vi "insert new subpanel.vi"(8 "error in":errorcluster, 9 "event":refnum<user-event>, 10 "mod data ref":refnum<data-value>, 11 "SubPanel in":refnum<vi>) -> (0 "error out":errorcluster, 3 "reference out":refnum<vi>)   [LabVIEW 2013, in "vi mod UI.lvlib"]
uses:
  vi mod UI.lvlib
  VI modification.lvclass
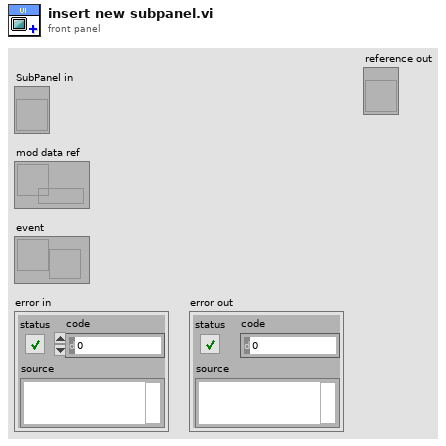
[diagram p1: front panel]
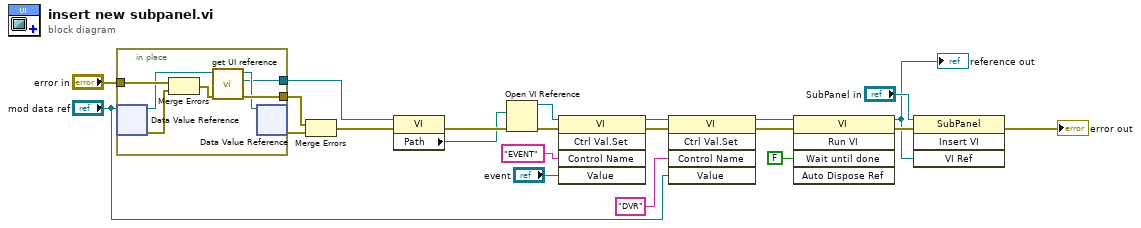
[diagram p0: block diagram]
diagram:
  n1 = in-place {
    in-place-border: "error in" -> [w29]
    in-place-border: [w28] -> w20
    in-place-border: [w23] -> w5
    n2 = in-place-dvr #1("mod data ref") -> (w27:refnum<class "VI modification.lvclass">, w24:errorcluster)
    n3 = Merge Errors(w29, w24) -> (w25:errorcluster)
    n4 = call-dynamic "get UI reference.vi"("error in"=w25, "VI modification in"=w27) -> ("error out"=w28:errorcluster, "VI Refnum"=w23:refnum<vi>, "VI modification out"=w26:refnum<class "VI modification.lvclass">)  [unwired: 7 in]
    n5 = in-place-dvr #1(w26) -> (w17:errorcluster)  [unwired: 1 out]
  }
  n6 = Merge Errors(w20, w17) -> (w18:errorcluster)
  n7 = property class="VI"(reference=w5, error in=w18) -> (error out=w7:errorcluster, "Path"=w4:path)  [unwired: 1 out]
  n8 = Open VI Reference(vi path=w4, error in (no error)=w7) -> (vi reference=w3:refnum<vi>, error out=w6:errorcluster)  [unwired: 4 in]
  n9 = invoke class="VI" method="Ctrl Val.Set"(reference=w3, error in=w6, "Control Name"="EVENT", "Value"="event") -> (reference out=w14:refnum<vi>, error out=w15:errorcluster)  [unwired: 1 in, 3 out]
  n10 = invoke class="VI" method="Ctrl Val.Set"(reference=w14, error in=w15, "Control Name"="DVR", "Value"="mod data ref") -> (reference out=w13:refnum<vi>, error out=w16:errorcluster)  [unwired: 1 in, 3 out]
  n11 = invoke class="VI" method="Run VI"(reference=w13, error in=w16, "Wait until done"=FALSE ("Wait Until Done")) -> (reference out=w2:refnum<vi>, error out=w19:errorcluster)  [unwired: 2 in, 3 out]
  "reference out" <- w2
  n12 = invoke on="Invoke Node" class="SubPanel" method="Insert VI"(reference="SubPanel in", error in=w19, "VI Ref"=w2) -> (error out=→"error out":errorcluster)  [unwired: 1 in, 3 out]
